vi "SUB_Write_GEN4_Init_data_V2_0_1.vi"(0 "Port-act 1":refnum<visa-resource-name>="COM8", 1 "data1":T7 {"Check sum" format="%x"; "Reserved_6" format="%x"; "Reserved_5" format="%x"; "Reserved_4" format="%x"; "Cal_Compart. A_10_4" format="%x"; "Reserved_3" format="%x"; "Reserved_2" format="%x"; "Reserved_1" format="%x"; "Cal_Compart. B_10_4" format="%x"; "Cal_Compart. B_10_3" format="%x"; "Cal_Compart. B_10_2" format="%x"; "Cal_Compart. B_10_1" format="%x"; "Cal_Compart. A_10_3" format="%x"; "Cal_Compart. A_10_2" format="%x"; "Cal_Compart. A_10_1" format="%x"; "Operative Side" format="%x"; "Firmware Revision" format="%x"; "Packet ID" format="%x"}, 2 "data2":T6 {"Check sum" format="%x"; "Cal_Compart. B_12_4" format="%x"; "Cal_Compart. B_12_3" format="%x"; "Cal_Compart. B_12_2" format="%x"; "Cal_Compart. B_11_2" format="%x"; "Cal_Compart. B_12_1" format="%x"; "Cal_Compart. A_12_4" format="%x"; "Cal_Compart. A_12_3" format="%x"; "Cal_Compart. A_12_2" format="%x"; "Cal_Compart. A_12_1" format="%x"; "Cal_Compart. B_11_4" format="%x"; "Cal_Compart. B_11_3" format="%x"; "Cal_Compart. B_11_1" format="%x"; "Cal_Compart. A_11_4" format="%x"; "Cal_Compart. A_11_3" format="%x"; "Cal_Compart. A_11_2" format="%x"; "Cal_Compart. A_11_1" format="%x"; "Packet ID" format="%x"}, 3 "Device information":T13 {"Check sum 2" format="%x"; "Device Type L" format="%x"; "Device Type H" format="%x"; "Check sum" format="%x"; "Scale B" format="%x"; "Scale A" format="%x"; "Manufacturer Lot ID 4" format="%x"; "Manufacturer Lot ID 3" format="%x"; "Manufacturer Lot ID 2" format="%x"; "Manufacturer Lot ID 1" format="%x"; "Day" format="%x"; "Month" format="%x"; "Year" format="%x"; "Device ID 4" format="%x"; "Device ID 3" format="%x"; "Device ID 2" format="%x"; "Device ID 1" format="%x"; "Packet ID" format="%x"}, 4 "Cal information":T12 {"Check sum" format="%x"; "Voltage L 2.8V" format="%x"; "Voltage H 2.8V" format="%x"; "Voltage L 3.1V" format="%x"; "Acc Z_L_Cal" format="%x"; "Voltage H 3.1V" format="%x"; "Gyro Z_L_Cal" format="%x"; "Gyro Z_H_Cal" format="%x"; "Gyro Y_L_Cal" format="%x"; "Gyro Y_H_Cal" format="%x"; "Gyro X_L_Cal" format="%x"; "Gyro X_H_Cal" format="%x"; "Acc Z_H_Cal" format="%x"; "Acc Y_L_Cal" format="%x"; "Acc Y_H_Cal" format="%x"; "Acc X_L_Cal" format="%x"; "Acc X_H_Cal" format="%x"; "Packet ID" format="%x"}, 5 "data3":T5 {"Check sum" format="%x"; "Cal_Compart. B_14_4" format="%x"; "Cal_Compart. B_14_3" format="%x"; "Cal_Compart. B_14_2" format="%x"; "Cal_Compart. B_13_2" format="%x"; "Cal_Compart. B_14_1" format="%x"; "Cal_Compart. A_14_4" format="%x"; "Cal_Compart. A_14_3" format="%x"; "Cal_Compart. A_14_2" format="%x"; "Cal_Compart. A_14_1" format="%x"; "Cal_Compart. B_13_4" format="%x"; "Cal_Compart. B_13_3" format="%x"; "Cal_Compart. B_13_1" format="%x"; "Cal_Compart. A_13_4" format="%x"; "Cal_Compart. A_13_3" format="%x"; "Cal_Compart. A_13_2" format="%x"; "Cal_Compart. A_13_1" format="%x"; "Packet ID" format="%x"}, 6 "data4":T4 {"Check sum" format="%x"; "Reserved_8" format="%x"; "Reserved_7" format="%x"; "Reserved_6" format="%x"; "Cal_Compart. B_16_2" format="%x"; "Reserved_5" format="%x"; "Reserved_4" format="%x"; "Reserved_3" format="%x"; "Reserved_2" format="%x"; "Reserved_1" format="%x"; "Cal_Compart. B_16_4" format="%x"; "Cal_Compart. B_16_3" format="%x"; "Cal_Compart. B_16_1" format="%x"; "Cal_Compart. A_16_4" format="%x"; "Cal_Compart. A_16_3" format="%x"; "Cal_Compart. A_16_2" format="%x"; "Cal_Compart. A_16_1" format="%x"; "Packet ID" format="%x"}, 7 "Connection Status":T8={"MAC Address"="F8:B8:54:EF:76:8D", "cnx handle"=0, "cnx flags"=5, "Address Type"=1, "Connection Interval (ms)"=8, "Timeout(ms)"=1000, "Latency"=0, "bonding handle"=255} {"Address Type" items=["Public", "Random"]}, 8 "Acclerometer value(0, 45)":T3 {"Check sum" format="%x"; "Reserved_4" format="%x"; "Reserved_3" format="%x"; "Reserved_2" format="%x"; "Acc. Z_0 val_L" format="%x"; "Reserved_1" format="%x"; "Acc. Z_45 val_L" format="%x"; "Acc. Z_45 val_H" format="%x"; "Acc. Y_45 val_L" format="%x"; "Acc. Y_45 val_H" format="%x"; "Acc. X_45 val_L" format="%x"; "Acc. X_45 val_H" format="%x"; "Acc. Z_0 val_H" format="%x"; "Acc. Y_0 val_L" format="%x"; "Acc. Y_0 val_H" format="%x"; "Acc. X_0 val_L" format="%x"; "Acc. X_0 val_H" format="%x"; "Packet ID" format="%x"}, 9 "Acclerometer value(90, 180)":T2 {"Check sum" format="%x"; "Reserved_2" format="%x"; "Reserved_1" format="%x"; "second counter_2" format="%x"; "Acc. Z_90 val_L" format="%x"; "second counter_1" format="%x"; "Acc. Z_180 val_L" format="%x"; "Acc. Z_180 val_H" format="%x"; "Acc. Y_180 val_L" format="%x"; "Acc. Y_180 val_H" format="%x"; "Acc. X_180 val_L" format="%x"; "Acc. X_180 val_H" format="%x"; "Acc. Z_90 val_H" format="%x"; "Acc. Y_90 val_L" format="%x"; "Acc. Y_90 val_H" format="%x"; "Acc. X_90 val_L" format="%x"; "Acc. X_90 val_H" format="%x"; "Packet ID" format="%x"}, 10 "배열":u8[](array[numeric]), 12 "Mode":T10, 13 "PCAP zero information":T11 {"Check sum" format="%x"; "Sensor 8_L" format="%x"; "Sensor 8_H" format="%x"; "Sensor 7_L" format="%x"; "Sensor 7_H" format="%x"; "Sensor 6_L" format="%x"; "Sensor 6_H" format="%x"; "Sensor 5_L" format="%x"; "Sensor 5_H" format="%x"; "Sensor 4_L" format="%x"; "Sensor 4_H" format="%x"; "Sensor 3_L" format="%x"; "Sensor 3_H" format="%x"; "Sensor 2_L" format="%x"; "Sensor 2_H" format="%x"; "Sensor 1_L" format="%x"; "Sensor 1_H" format="%x"; "Packet ID" format="%x"}, 14 "Interval Time":enum16{"10ms", "33ms", "50ms"}(ring)) -> (27 "불리언":bool)   [LabVIEW 2015]
uses:
  Cluster Type/Device information.ctl
  Cluster Type/Cal information.ctl
  Cluster Type/PCAP zero information.ctl
  Type definition/write_mode.ctl
  Lib_Bled112 toolkit/type_def/connection_status_bundle.ctl
  Lib_Bled112 toolkit/type_def/address_type.ctl
  Cluster Type/add data1.ctl
  Cluster Type/add data2.ctl
  Cluster Type/add data3.ctl
  Cluster Type/add data4.ctl
  Cluster Type/Acclerometer value(0, 45).ctl
  Cluster Type/Acclerometer value(90, 180).ctl
  Lib_Bled112 toolkit/ble_functions/ble_write_by_handle_uint8array.vi
panel:
  in  "열거형":T1(ring)
  in  "Delay(ms)":u32=3
  # "(Device Type is divided 1byte)"
  # "=> Sensor Offset Valure"
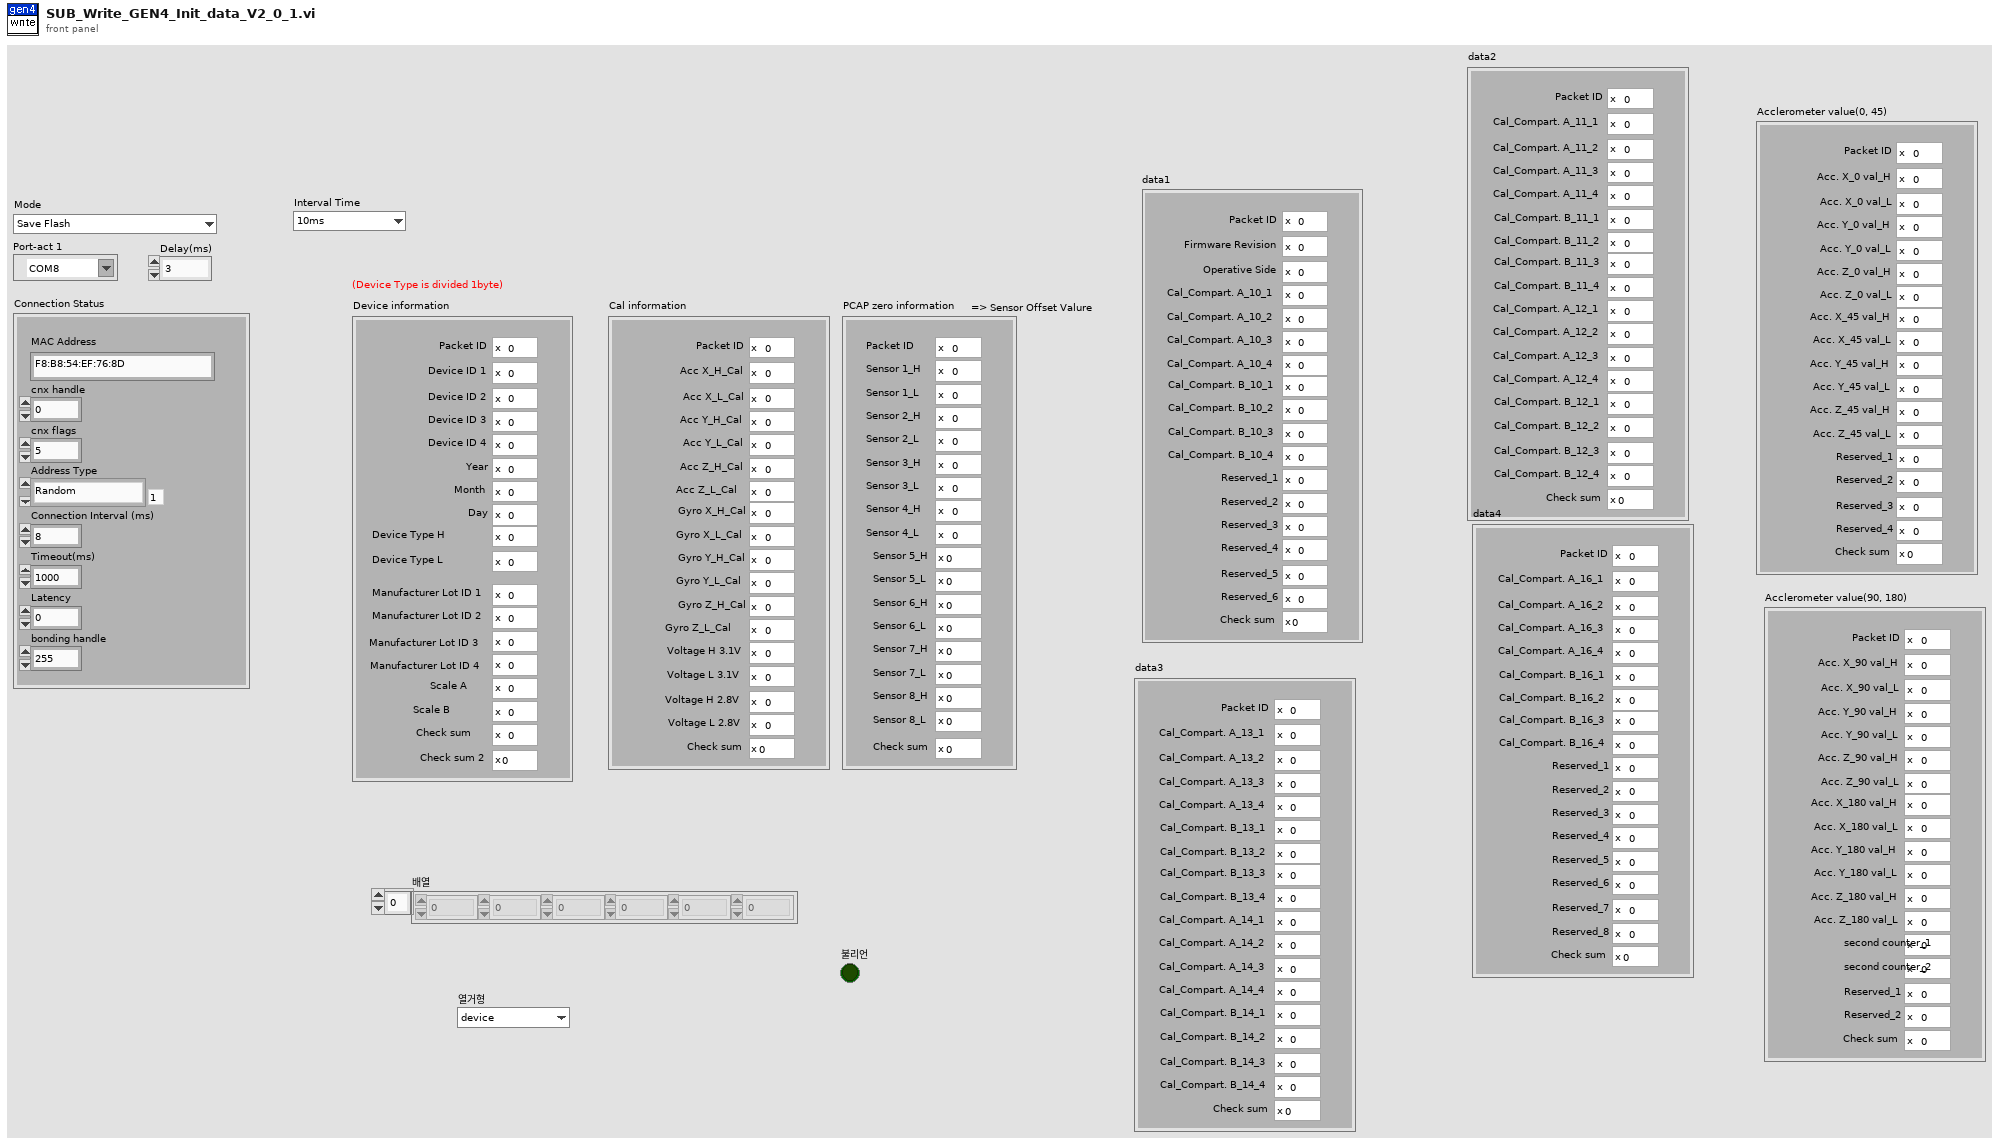
[diagram p1: front panel]
types:
  T1 = enum16{"device", "cal infor", "pcap", "data1", "data2", "data3", "data4", "acc 0", "acc 90", "42"}
  T2 = typedef "Acclerometer value(90, 180).ctl" = cluster{"Packet ID":u8, "Acc. X_90 val_H":u8, "Acc. X_90 val_L":u8, "Acc. Y_90 val_H":u8, "Acc. Y_90 val_L":u8, "Acc. Z_90 val_H":u8, "Acc. Z_90 val_L":u8, "Acc. X_180 val_H":u8, "Acc. X_180 val_L":u8, "Acc. Y_180 val_H":u8, "Acc. Y_180 val_L":u8, "Acc. Z_180 val_H":u8, "Acc. Z_180 val_L":u8, "second counter_1":u8, "second counter_2":u8, "Reserved_1":u8, "Reserved_2":u8, "Check sum":u8}
  T3 = typedef "Acclerometer value(0, 45).ctl" = cluster{"Packet ID":u8, "Acc. X_0 val_H":u8, "Acc. X_0 val_L":u8, "Acc. Y_0 val_H":u8, "Acc. Y_0 val_L":u8, "Acc. Z_0 val_H":u8, "Acc. Z_0 val_L":u8, "Acc. X_45 val_H":u8, "Acc. X_45 val_L":u8, "Acc. Y_45 val_H":u8, "Acc. Y_45 val_L":u8, "Acc. Z_45 val_H":u8, "Acc. Z_45 val_L":u8, "Reserved_1":u8, "Reserved_2":u8, "Reserved_3":u8, "Reserved_4":u8, "Check sum":u8}
  T4 = typedef "add data4.ctl" = cluster{"Packet ID":u8, "Cal_Compart. A_16_1":u8, "Cal_Compart. A_16_2":u8, "Cal_Compart. A_16_3":u8, "Cal_Compart. A_16_4":u8, "Cal_Compart. B_16_1":u8, "Cal_Compart. B_16_2":u8, "Cal_Compart. B_16_3":u8, "Cal_Compart. B_16_4":u8, "Reserved_1":u8, "Reserved_2":u8, "Reserved_3":u8, "Reserved_4":u8, "Reserved_5":u8, "Reserved_6":u8, "Reserved_7":u8, "Reserved_8":u8, "Check sum":u8}
  T5 = typedef "add data3.ctl" = cluster{"Packet ID":u8, "Cal_Compart. A_13_1":u8, "Cal_Compart. A_13_2":u8, "Cal_Compart. A_13_3":u8, "Cal_Compart. A_13_4":u8, "Cal_Compart. B_13_1":u8, "Cal_Compart. B_13_2":u8, "Cal_Compart. B_13_3":u8, "Cal_Compart. B_13_4":u8, "Cal_Compart. A_14_1":u8, "Cal_Compart. A_14_2":u8, "Cal_Compart. A_14_3":u8, "Cal_Compart. A_14_4":u8, "Cal_Compart. B_14_1":u8, "Cal_Compart. B_14_2":u8, "Cal_Compart. B_14_3":u8, "Cal_Compart. B_14_4":u8, "Check sum":u8}
  T6 = typedef "add data2.ctl" = cluster{"Packet ID":u8, "Cal_Compart. A_11_1":u8, "Cal_Compart. A_11_2":u8, "Cal_Compart. A_11_3":u8, "Cal_Compart. A_11_4":u8, "Cal_Compart. B_11_1":u8, "Cal_Compart. B_11_2":u8, "Cal_Compart. B_11_3":u8, "Cal_Compart. B_11_4":u8, "Cal_Compart. A_12_1":u8, "Cal_Compart. A_12_2":u8, "Cal_Compart. A_12_3":u8, "Cal_Compart. A_12_4":u8, "Cal_Compart. B_12_1":u8, "Cal_Compart. B_12_2":u8, "Cal_Compart. B_12_3":u8, "Cal_Compart. B_12_4":u8, "Check sum":u8}
  T7 = typedef "add data1.ctl" = cluster{"Packet ID":u8, "Firmware Revision":u8, "Operative Side":u8, "Cal_Compart. A_10_1":u8, "Cal_Compart. A_10_2":u8, "Cal_Compart. A_10_3":u8, "Cal_Compart. A_10_4":u8, "Cal_Compart. B_10_1":u8, "Cal_Compart. B_10_2":u8, "Cal_Compart. B_10_3":u8, "Cal_Compart. B_10_4":u8, "Reserved_1":u8, "Reserved_2":u8, "Reserved_3":u8, "Reserved_4":u8, "Reserved_5":u8, "Reserved_6":u8, "Check sum":u8}
  T8 = typedef "connection_status_bundle.ctl" = cluster{"MAC Address":string, "cnx handle":u8, "cnx flags":u8, "Address Type":T9, "Connection Interval (ms)":u16, "Timeout(ms)":u16, "Latency":u16, "bonding handle":u8}
  T9 = typedef "address_type.ctl" = u8
  T10 = typedef "write_mode.ctl" = enum16{"Save Flash", "Visa save", "Interval Change"}
  T11 = typedef "PCAP zero information.ctl" = cluster{"Packet ID":u8, "Sensor 1_H":u8, "Sensor 1_L":u8, "Sensor 2_H":u8, "Sensor 2_L ":u8, "Sensor 3_H":u8, "Sensor 3_L":u8, "Sensor 4_H":u8, "Sensor 4_L":u8, "Sensor 5_H":u8, "Sensor 5_L":u8, "Sensor 6_H":u8, "Sensor 6_L":u8, "Sensor 7_H":u8, "Sensor 7_L":u8, "Sensor 8_H":u8, "Sensor 8_L":u8, "Check sum":u8}
  T12 = typedef "Cal information.ctl" = cluster{"Packet ID":u8, "Acc X_H_Cal":u8, "Acc X_L_Cal":u8, "Acc Y_H_Cal":u8, "Acc Y_L_Cal":u8, "Acc Z_H_Cal":u8, "Acc Z_L_Cal":u8, "Gyro X_H_Cal":u8, "Gyro X_L_Cal":u8, "Gyro Y_H_Cal":u8, "Gyro Y_L_Cal":u8, "Gyro Z_H_Cal":u8, "Gyro Z_L_Cal":u8, "Voltage H 3.1V":u8, "Voltage L 3.1V":u8, "Voltage H 2.8V":u8, "Voltage L 2.8V":u8, "Check sum":u8}
  T13 = typedef "Device information.ctl" = cluster{"Packet ID":u8, "Device ID 1":u8, "Device ID 2":u8, "Device ID 3":u8, "Device ID 4":u8, "Year":u8, "Month":u8, "Day":u8, "Device Type H":u8, "Device Type L":u8, "Manufacturer Lot ID 1":u8, "Manufacturer Lot ID 2":u8, "Manufacturer Lot ID 3":u8, "Manufacturer Lot ID 4":u8, "Scale A":u8, "Scale B":u8, "Check sum":u8, "Check sum 2":u8}
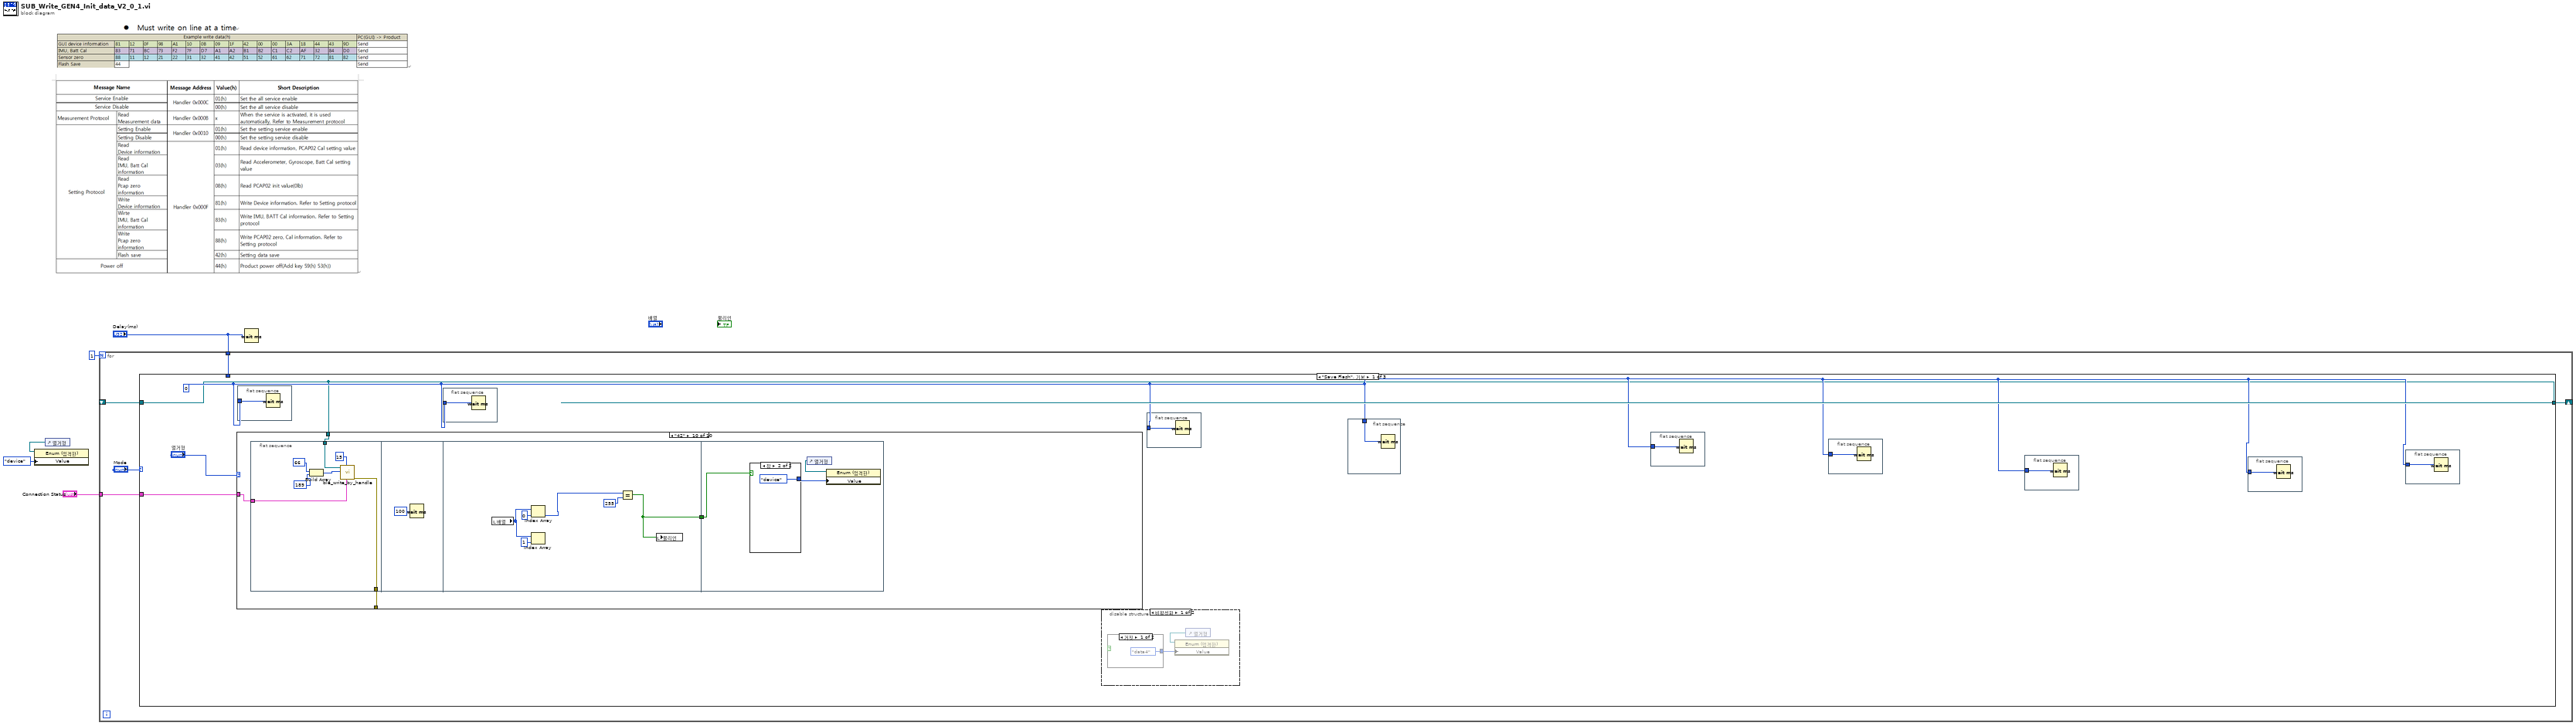
[diagram p0: block diagram]
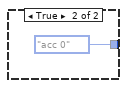
[diagram p2: hidden frame]
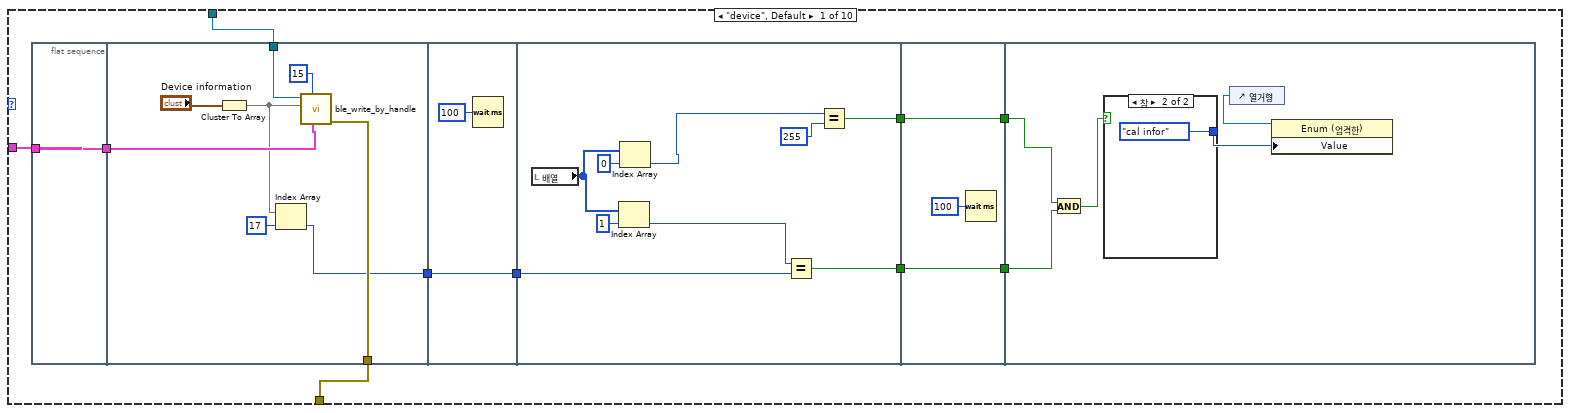
[diagram p4: hidden frame]
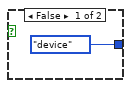
[diagram p5: hidden frame]
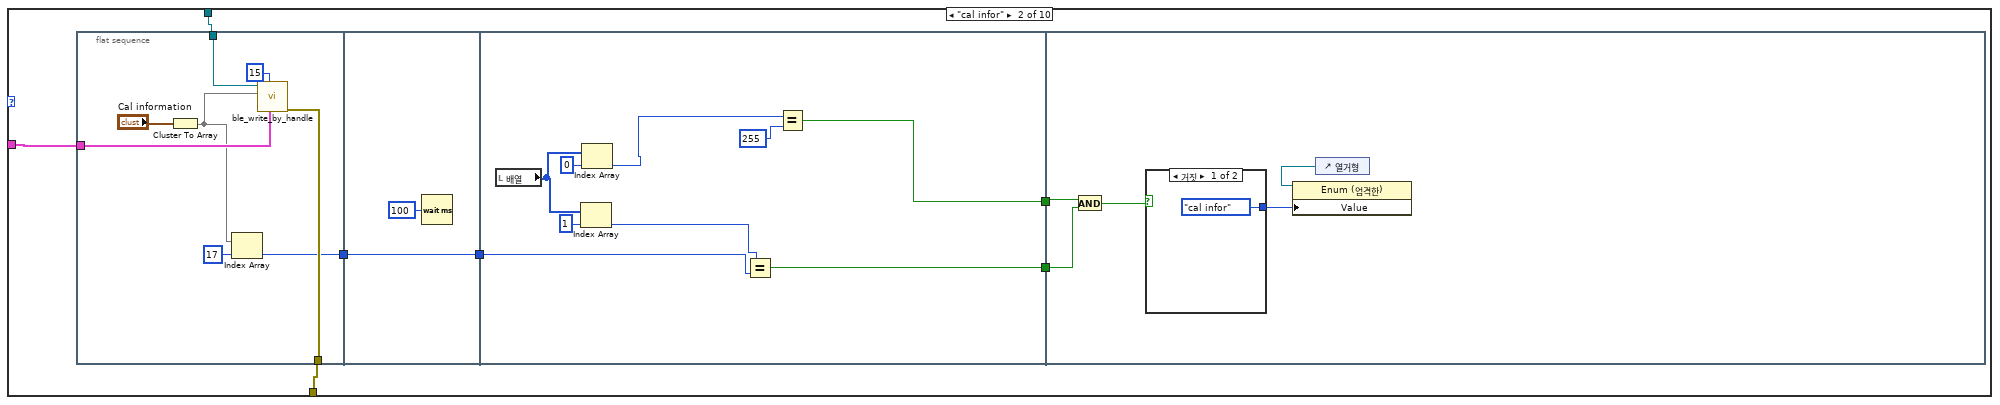
[diagram p6: hidden frame]
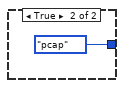
[diagram p7: hidden frame]
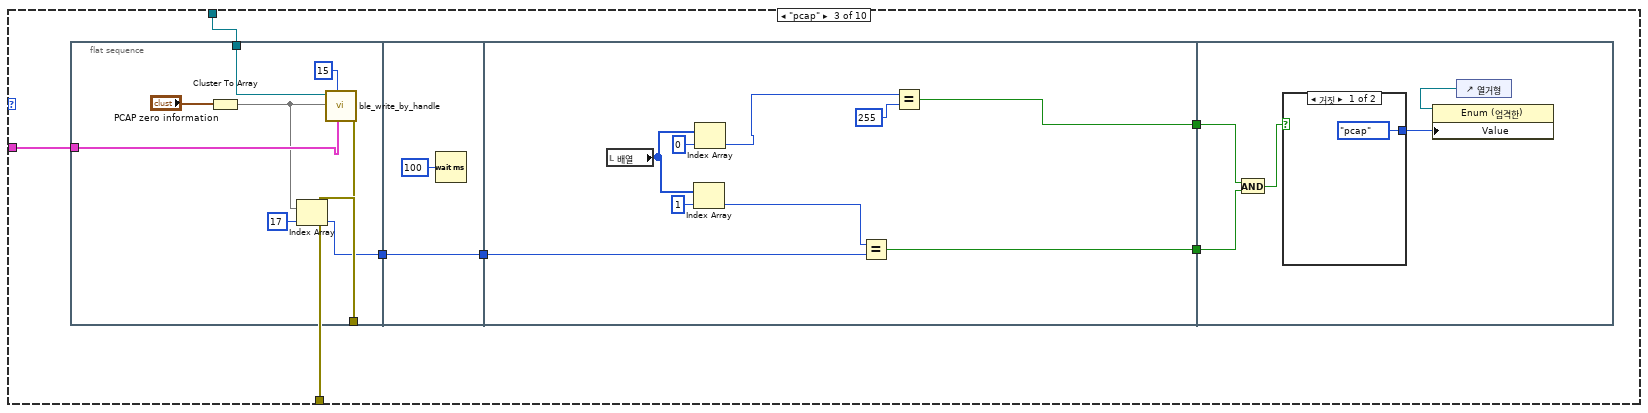
[diagram p8: hidden frame]
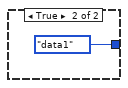
[diagram p9: hidden frame]
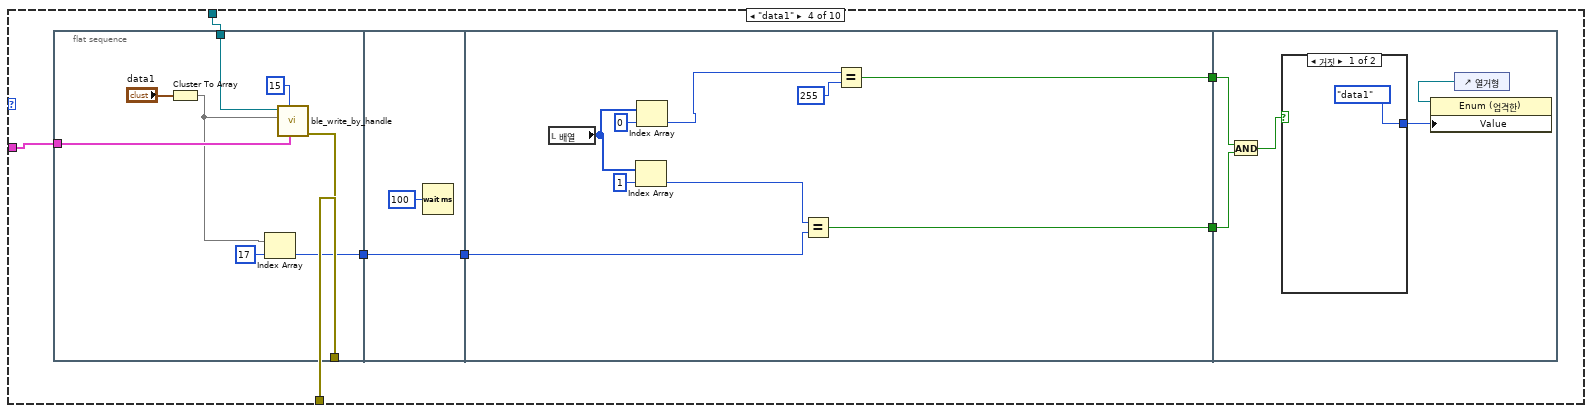
[diagram p10: hidden frame]
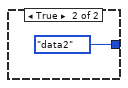
[diagram p11: hidden frame]
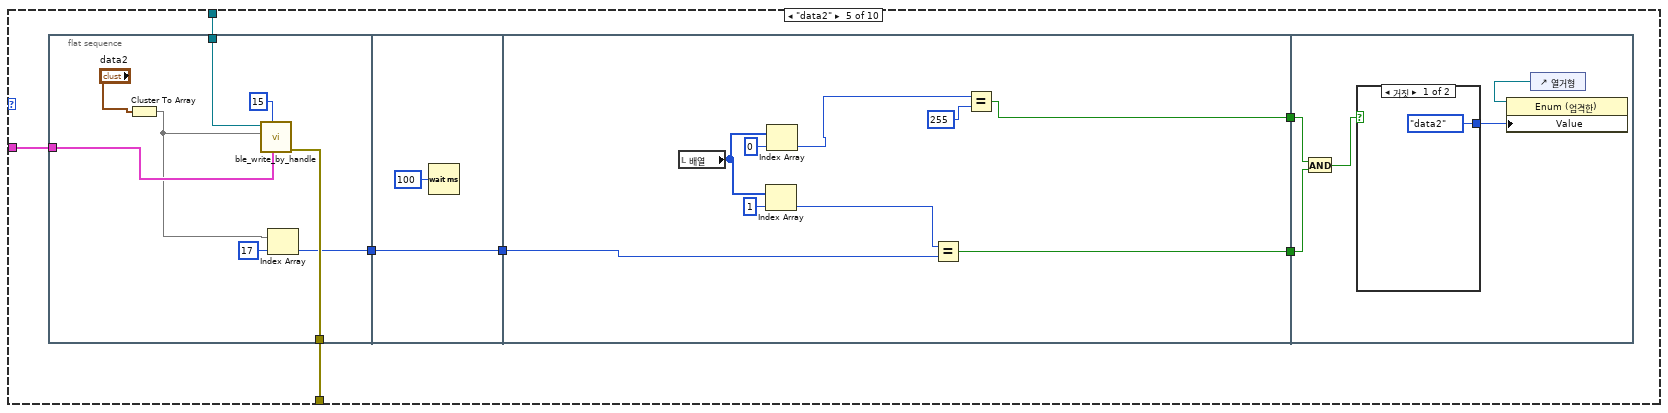
[diagram p12: hidden frame]
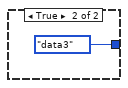
[diagram p13: hidden frame]
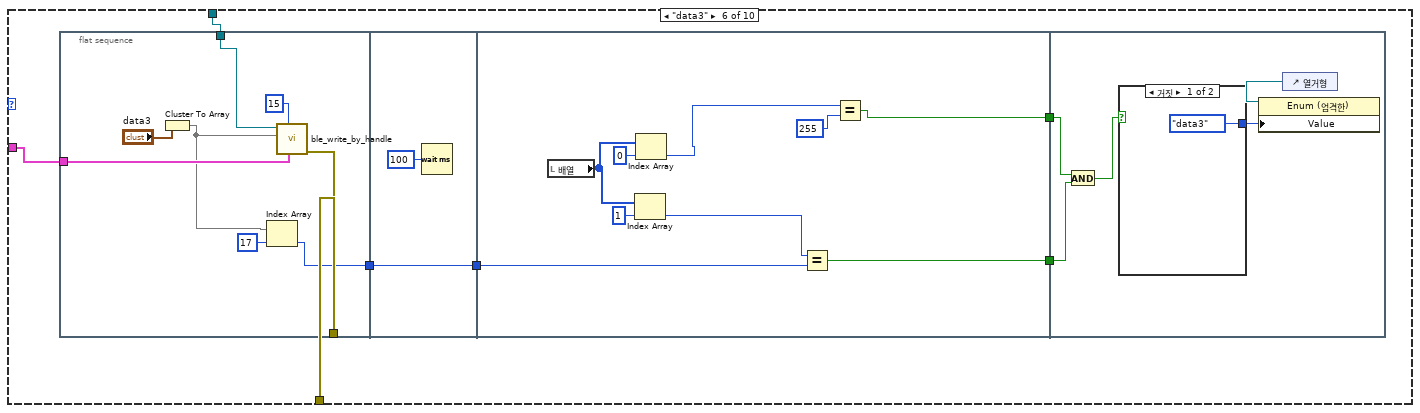
[diagram p14: hidden frame]
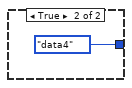
[diagram p15: hidden frame]
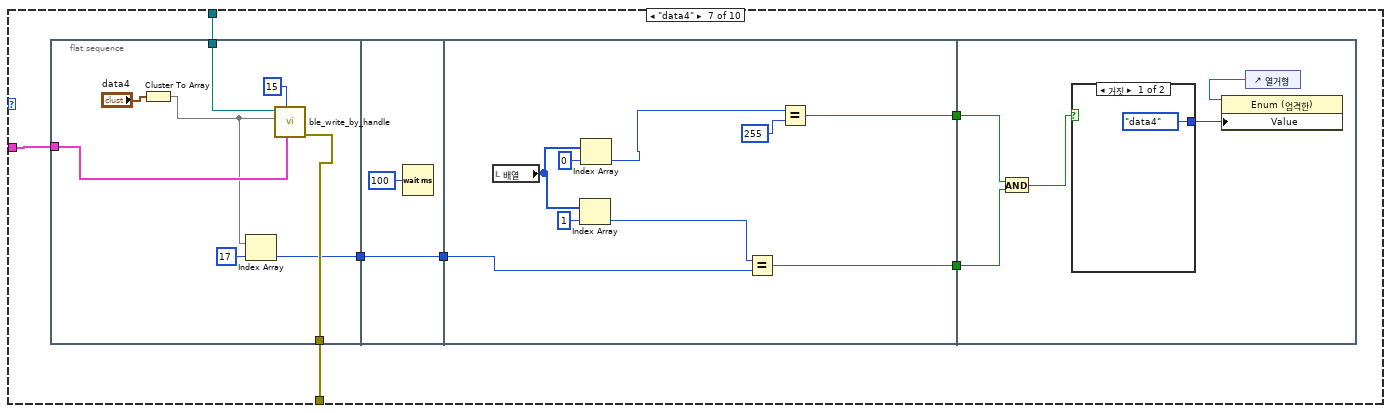
[diagram p16: hidden frame]
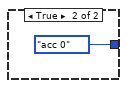
[diagram p17: hidden frame]
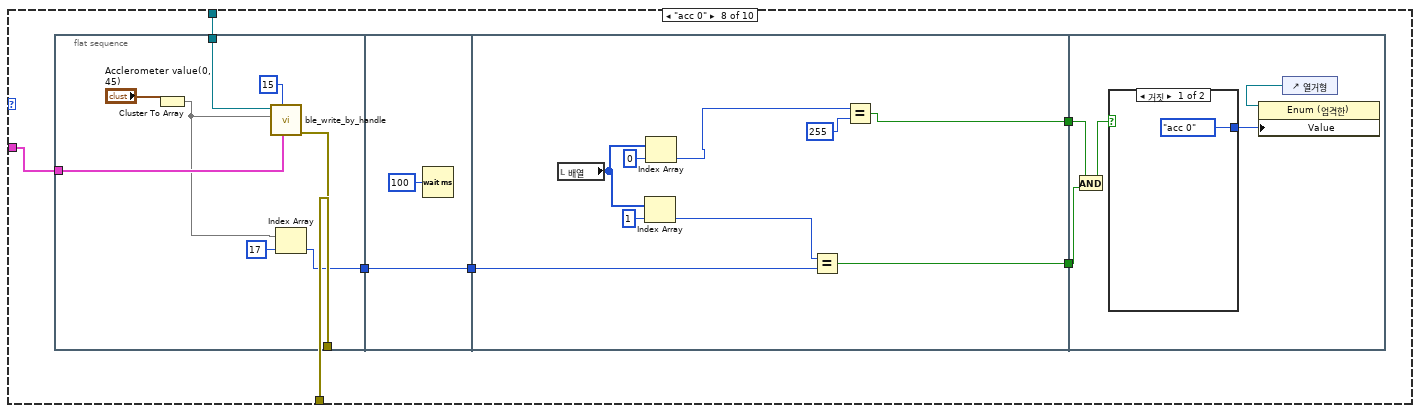
[diagram p18: hidden frame]
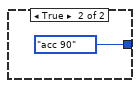
[diagram p19: hidden frame]
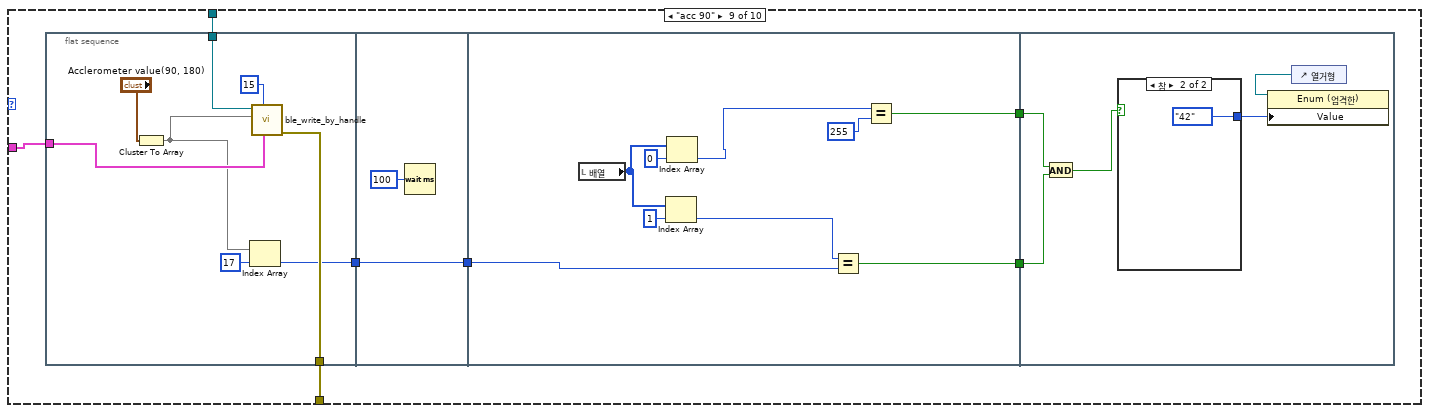
[diagram p20: hidden frame]
diagram:
  n1 = control-ref of="열거형"() -> (w1:refnum<vi>)
  n2 = property class="Enum (엄격한)"(reference=w1, "Value"=T1."device" ("값")) -> ()  [unwired: 1 in, 2 out]
  n3 = for {
    N: 1 -> [_]
    shift-right: [w9] -> _
    shift-left: _ -> [w8]
    tunnel: "Connection Status" -> [w7]
    tunnel: "Delay(ms)" -> [w6]
    n4 = case shown="\"Save Flash\", 기본" "Mode" {
      tunnel: [w11 w372 "Port-act 1"] -> w9
      tunnel: w8 -> [w11 w372 _]
      tunnel: w7 -> [w12 w385 _]
      tunnel: w6 -> [_ w360 _]
      frame "Save Flash", Default {
        w14 = u32 0 ("대기 시간(ms)")
        n5 = case shown="\"42\"" "열거형" {
          tunnel: w12 -> [w28 w64 w98 w130 w164 w196 w230 w263 w296 w326]
          tunnel: w11 -> [w27 w65 w97 w131 w163 w197 w229 w262 w295 w325]
          tunnel: [w26 w63 w96 w129 w162 w195 w228 w261 w294 w324] -> _
          frame "device", Default {
            n6 = flat-sequence {
              tunnel: w28 -> [w29]
              tunnel: [w29] -> w25
              tunnel: w27 -> [w34]
              tunnel: [w33] -> w26
              tunnel: w25 -> [w35]
              tunnel: [w30] -> w22
              tunnel: w22 -> [w38]
              tunnel: [w38] -> w21
              tunnel: [w43] -> w24
              tunnel: w21 -> [w41]
              tunnel: [w40] -> w20
              tunnel: w24 -> [w51]
              tunnel: [w51] -> w23
              tunnel: w20 -> [w49]
              tunnel: [w49] -> w19
              tunnel: w23 -> [w54]
              tunnel: w19 -> [w53]
              frame #0 {
              }
              frame #1 {
                n7 = Cluster To Array(cluster="Device information") -> (array=w31:u8[])
                n8 = Index Array(array=w31, index=17 ("인덱스")) -> (element=w30:u8)
                n9 = call-poly "ble_write_by_handle.vi"("Connection Status"=w35, "Handle"=u16 15, "data (uint8array)"=w31, "COM Bluegiga in"=w34) -> ("error out"=w33:errorcluster)  [unwired: 6 in, 1 out]
              }
              frame #2 {
                n10 = Wait (ms)(milliseconds to wait=u32 100 ("대기 시간(ms)")) -> ()  [unwired: 1 out]
              }
              frame #3 {
                n11 = local read "배열"() -> (w44:u8[])
                n12 = Index Array(array=w44, index=1 ("인덱스")) -> (element=w42:u8)
                n13 = Index Array(array=w44, index=0 ("인덱스")) -> (element=w47:u8)
                n14 = Equal?(x=w42, y=w41) -> (x = y?=w40:bool)
                n15 = Equal?(x=w47, y=u8 255) -> (x = y?=w43:bool)
              }
              frame #4 {
                n16 = Wait (ms)(milliseconds to wait=u32 100 ("대기 시간(ms)")) -> ()  [unwired: 1 out]
              }
              frame #5 {
                n17 = And(x=w54, y=w53) -> (x .and. y?=w52:bool)
                n18 = case shown="참" w52 {
                  tunnel: [T1."device" ("값") T1."cal infor" ("값")] -> w55
                  frame False {
                  }
                  frame True {
                  }
                }
                n19 = control-ref of="열거형"() -> (w56:refnum<vi>)
                n20 = property class="Enum (엄격한)"(reference=w56, "Value"=w55) -> ()  [unwired: 1 in, 2 out]
              }
            }
          }
          frame "cal infor" {
            n21 = flat-sequence {
              tunnel: w65 -> [w71]
              tunnel: w64 -> [w70]
              tunnel: [w69] -> w63
              tunnel: [w66] -> w61
              tunnel: w61 -> [w74]
              tunnel: [w74] -> w60
              tunnel: [w79] -> w62
              tunnel: w60 -> [w78]
              tunnel: [w76] -> w59
              tunnel: w62 -> [w87]
              tunnel: w59 -> [w86]
              frame #0 {
                n22 = Cluster To Array(cluster="Cal information") -> (array=w67:u8[])
                n23 = Index Array(array=w67, index=17 ("인덱스")) -> (element=w66:u8)
                n24 = call-poly "ble_write_by_handle.vi"("Connection Status"=w70, "Handle"=u16 15, "data (uint8array)"=w67, "COM Bluegiga in"=w71) -> ("error out"=w69:errorcluster)  [unwired: 6 in, 1 out]
              }
              frame #1 {
                n25 = Wait (ms)(milliseconds to wait=u32 100 ("대기 시간(ms)")) -> ()  [unwired: 1 out]
              }
              frame #2 {
                n26 = local read "배열"() -> (w80:u8[])
                n27 = Index Array(array=w80, index=1 ("인덱스")) -> (element=w77:u8)
                n28 = Index Array(array=w80, index=0 ("인덱스")) -> (element=w83:u8)
                n29 = Equal?(x=w77, y=w78) -> (x = y?=w76:bool)
                n30 = Equal?(x=w83, y=u8 255) -> (x = y?=w79:bool)
              }
              frame #3 {
                n31 = And(x=w87, y=w86) -> (x .and. y?=w85:bool)
                n32 = case shown="거짓" w85 {
                  tunnel: [T1."cal infor" ("값") T1."pcap" ("값")] -> w88
                  frame False {
                  }
                  frame True {
                  }
                }
                n33 = control-ref of="열거형"() -> (w89:refnum<vi>)
                n34 = property class="Enum (엄격한)"(reference=w89, "Value"=w88) -> ()  [unwired: 1 in, 2 out]
              }
            }
          }
          frame "pcap" {
            n35 = flat-sequence {
              tunnel: w98 -> [w104]
              tunnel: w97 -> [w103]
              tunnel: [w102] -> w96
              tunnel: [w99] -> w94
              tunnel: w94 -> [w107]
              tunnel: [w107] -> w93
              tunnel: [w112] -> w95
              tunnel: w93 -> [w110]
              tunnel: [w109] -> w92
              tunnel: w95 -> [w120]
              tunnel: w92 -> [w119]
              frame #0 {
                n36 = Cluster To Array(cluster="PCAP zero information") -> (array=w100:u8[])
                n37 = Index Array(array=w100, index=17 ("인덱스")) -> (element=w99:u8)
                n38 = call-poly "ble_write_by_handle.vi"("Connection Status"=w104, "Handle"=u16 15, "data (uint8array)"=w100, "COM Bluegiga in"=w103) -> ("error out"=w102:errorcluster)  [unwired: 6 in, 1 out]
              }
              frame #1 {
                n39 = Wait (ms)(milliseconds to wait=u32 100 ("대기 시간(ms)")) -> ()  [unwired: 1 out]
              }
              frame #2 {
                n40 = local read "배열"() -> (w113:u8[])
                n41 = Index Array(array=w113, index=1 ("인덱스")) -> (element=w111:u8)
                n42 = Index Array(array=w113, index=0 ("인덱스")) -> (element=w116:u8)
                n43 = Equal?(x=w111, y=w110) -> (x = y?=w109:bool)
                n44 = Equal?(x=w116, y=u8 255) -> (x = y?=w112:bool)
              }
              frame #3 {
                n45 = And(x=w120, y=w119) -> (x .and. y?=w118:bool)
                n46 = case shown="거짓" w118 {
                  tunnel: [T1."pcap" ("값") T1."data1" ("값")] -> w121
                  frame False {
                  }
                  frame True {
                  }
                }
                n47 = control-ref of="열거형"() -> (w122:refnum<vi>)
                n48 = property class="Enum (엄격한)"(reference=w122, "Value"=w121) -> ()  [unwired: 1 in, 2 out]
              }
            }
          }
          frame "data1" {
            n49 = flat-sequence {
              tunnel: w131 -> [w137]
              tunnel: w130 -> [w136]
              tunnel: [w135] -> w129
              tunnel: [w132] -> w127
              tunnel: w127 -> [w140]
              tunnel: [w140] -> w126
              tunnel: [w145] -> w128
              tunnel: w126 -> [w144]
              tunnel: [w142] -> w125
              tunnel: w128 -> [w153]
              tunnel: w125 -> [w152]
              frame #0 {
                n50 = Cluster To Array(cluster="data1") -> (array=w133:u8[])
                n51 = Index Array(array=w133, index=17 ("인덱스")) -> (element=w132:u8)
                n52 = call-poly "ble_write_by_handle.vi"("Connection Status"=w136, "Handle"=u16 15, "data (uint8array)"=w133, "COM Bluegiga in"=w137) -> ("error out"=w135:errorcluster)  [unwired: 6 in, 1 out]
              }
              frame #1 {
                n53 = Wait (ms)(milliseconds to wait=u32 100 ("대기 시간(ms)")) -> ()  [unwired: 1 out]
              }
              frame #2 {
                n54 = local read "배열"() -> (w146:u8[])
                n55 = Index Array(array=w146, index=1 ("인덱스")) -> (element=w143:u8)
                n56 = Index Array(array=w146, index=0 ("인덱스")) -> (element=w149:u8)
                n57 = Equal?(x=w143, y=w144) -> (x = y?=w142:bool)
                n58 = Equal?(x=w149, y=u8 255) -> (x = y?=w145:bool)
              }
              frame #3 {
                n59 = And(x=w153, y=w152) -> (x .and. y?=w151:bool)
                n60 = case shown="거짓" w151 {
                  tunnel: [T1."data1" ("값") T1."data2" ("값")] -> w154
                  frame False {
                  }
                  frame True {
                  }
                }
                n61 = control-ref of="열거형"() -> (w155:refnum<vi>)
                n62 = property class="Enum (엄격한)"(reference=w155, "Value"=w154) -> ()  [unwired: 1 in, 2 out]
              }
            }
          }
          frame "data2" {
            n63 = flat-sequence {
              tunnel: w164 -> [w170]
              tunnel: w163 -> [w169]
              tunnel: [w168] -> w162
              tunnel: [w165] -> w160
              tunnel: w160 -> [w173]
              tunnel: [w173] -> w159
              tunnel: [w178] -> w161
              tunnel: w159 -> [w176]
              tunnel: [w175] -> w158
              tunnel: w161 -> [w186]
              tunnel: w158 -> [w185]
              frame #0 {
                n64 = Cluster To Array(cluster="data2") -> (array=w166:u8[])
                n65 = call-poly "ble_write_by_handle.vi"("Connection Status"=w170, "Handle"=u16 15, "data (uint8array)"=w166, "COM Bluegiga in"=w169) -> ("error out"=w168:errorcluster)  [unwired: 6 in, 1 out]
                n66 = Index Array(array=w166, index=17 ("인덱스")) -> (element=w165:u8)
              }
              frame #1 {
                n67 = Wait (ms)(milliseconds to wait=u32 100 ("대기 시간(ms)")) -> ()  [unwired: 1 out]
              }
              frame #2 {
                n68 = local read "배열"() -> (w179:u8[])
                n69 = Index Array(array=w179, index=1 ("인덱스")) -> (element=w177:u8)
                n70 = Index Array(array=w179, index=0 ("인덱스")) -> (element=w182:u8)
                n71 = Equal?(x=w177, y=w176) -> (x = y?=w175:bool)
                n72 = Equal?(x=w182, y=u8 255) -> (x = y?=w178:bool)
              }
              frame #3 {
                n73 = And(x=w186, y=w185) -> (x .and. y?=w184:bool)
                n74 = case shown="거짓" w184 {
                  tunnel: [T1."data2" ("값") T1."data3" ("값")] -> w187
                  frame False {
                  }
                  frame True {
                  }
                }
                n75 = control-ref of="열거형"() -> (w188:refnum<vi>)
                n76 = property class="Enum (엄격한)"(reference=w188, "Value"=w187) -> ()  [unwired: 1 in, 2 out]
              }
            }
          }
          frame "data3" {
            n77 = flat-sequence {
              tunnel: w197 -> [w203]
              tunnel: w196 -> [w202]
              tunnel: [w201] -> w195
              tunnel: [w198] -> w193
              tunnel: w193 -> [w206]
              tunnel: [w206] -> w192
              tunnel: [w211] -> w194
              tunnel: w192 -> [w209]
              tunnel: [w208] -> w191
              tunnel: w194 -> [w219]
              tunnel: w191 -> [w218]
              frame #0 {
                n78 = Cluster To Array(cluster="data3") -> (array=w199:u8[])
                n79 = Index Array(array=w199, index=17 ("인덱스")) -> (element=w198:u8)
                n80 = call-poly "ble_write_by_handle.vi"("Connection Status"=w202, "Handle"=u16 15, "data (uint8array)"=w199, "COM Bluegiga in"=w203) -> ("error out"=w201:errorcluster)  [unwired: 6 in, 1 out]
              }
              frame #1 {
                n81 = Wait (ms)(milliseconds to wait=u32 100 ("대기 시간(ms)")) -> ()  [unwired: 1 out]
              }
              frame #2 {
                n82 = local read "배열"() -> (w212:u8[])
                n83 = Index Array(array=w212, index=1 ("인덱스")) -> (element=w210:u8)
                n84 = Index Array(array=w212, index=0 ("인덱스")) -> (element=w215:u8)
                n85 = Equal?(x=w210, y=w209) -> (x = y?=w208:bool)
                n86 = Equal?(x=w215, y=u8 255) -> (x = y?=w211:bool)
              }
              frame #3 {
                n87 = And(x=w219, y=w218) -> (x .and. y?=w217:bool)
                n88 = case shown="거짓" w217 {
                  tunnel: [T1."data3" ("값") T1."data4" ("값")] -> w220
                  frame False {
                  }
                  frame True {
                  }
                }
                n89 = control-ref of="열거형"() -> (w221:refnum<vi>)
                n90 = property class="Enum (엄격한)"(reference=w221, "Value"=w220) -> ()  [unwired: 1 in, 2 out]
              }
            }
          }
          frame "data4" {
            n91 = flat-sequence {
              tunnel: w230 -> [w236]
              tunnel: w229 -> [w235]
              tunnel: [w234] -> w228
              tunnel: [w232] -> w226
              tunnel: w226 -> [w239]
              tunnel: [w239] -> w225
              tunnel: [w244] -> w227
              tunnel: w225 -> [w242]
              tunnel: [w241] -> w224
              tunnel: w227 -> [w252]
              tunnel: w224 -> [w251]
              frame #0 {
                n92 = Cluster To Array(cluster="data4") -> (array=w231:u8[])
                n93 = Index Array(array=w231, index=17 ("인덱스")) -> (element=w232:u8)
                n94 = call-poly "ble_write_by_handle.vi"("Connection Status"=w236, "Handle"=u16 15, "data (uint8array)"=w231, "COM Bluegiga in"=w235) -> ("error out"=w234:errorcluster)  [unwired: 6 in, 1 out]
              }
              frame #1 {
                n95 = Wait (ms)(milliseconds to wait=u32 100 ("대기 시간(ms)")) -> ()  [unwired: 1 out]
              }
              frame #2 {
                n96 = local read "배열"() -> (w245:u8[])
                n97 = Index Array(array=w245, index=1 ("인덱스")) -> (element=w243:u8)
                n98 = Index Array(array=w245, index=0 ("인덱스")) -> (element=w248:u8)
                n99 = Equal?(x=w243, y=w242) -> (x = y?=w241:bool)
                n100 = Equal?(x=w248, y=u8 255) -> (x = y?=w244:bool)
              }
              frame #3 {
                n101 = And(x=w252, y=w251) -> (x .and. y?=w250:bool)
                n102 = case shown="거짓" w250 {
                  tunnel: [T1."data4" ("값") T1."acc 0" ("값")] -> w253
                  frame False {
                  }
                  frame True {
                  }
                }
                n103 = control-ref of="열거형"() -> (w254:refnum<vi>)
                n104 = property class="Enum (엄격한)"(reference=w254, "Value"=w253) -> ()  [unwired: 1 in, 2 out]
              }
            }
          }
          frame "acc 0" {
            n105 = flat-sequence {
              tunnel: w263 -> [w269]
              tunnel: w262 -> [w268]
              tunnel: [w267] -> w261
              tunnel: [w265] -> w259
              tunnel: w259 -> [w272]
              tunnel: [w272] -> w258
              tunnel: [w277] -> w260
              tunnel: w258 -> [w275]
              tunnel: [w274] -> w257
              tunnel: w260 -> [w285]
              tunnel: w257 -> [w284]
              frame #0 {
                n106 = Cluster To Array(cluster="Acclerometer value(0, 45)") -> (array=w264:u8[])
                n107 = call-poly "ble_write_by_handle.vi"("Connection Status"=w269, "Handle"=u16 15, "data (uint8array)"=w264, "COM Bluegiga in"=w268) -> ("error out"=w267:errorcluster)  [unwired: 6 in, 1 out]
                n108 = Index Array(array=w264, index=17 ("인덱스")) -> (element=w265:u8)
              }
              frame #1 {
                n109 = Wait (ms)(milliseconds to wait=u32 100 ("대기 시간(ms)")) -> ()  [unwired: 1 out]
              }
              frame #2 {
                n110 = local read "배열"() -> (w278:u8[])
                n111 = Index Array(array=w278, index=1 ("인덱스")) -> (element=w276:u8)
                n112 = Index Array(array=w278, index=0 ("인덱스")) -> (element=w281:u8)
                n113 = Equal?(x=w276, y=w275) -> (x = y?=w274:bool)
                n114 = Equal?(x=w281, y=u8 255) -> (x = y?=w277:bool)
              }
              frame #3 {
                n115 = And(x=w285, y=w284) -> (x .and. y?=w283:bool)
                n116 = case shown="거짓" w283 {
                  tunnel: [T1."acc 0" ("값") T1."acc 90" ("값")] -> w286
                  frame False {
                  }
                  frame True {
                  }
                }
                n117 = control-ref of="열거형"() -> (w287:refnum<vi>)
                n118 = property class="Enum (엄격한)"(reference=w287, "Value"=w286) -> ()  [unwired: 1 in, 2 out]
              }
            }
          }
          frame "acc 90" {
            n119 = flat-sequence {
              tunnel: w296 -> [w302]
              tunnel: w295 -> [w301]
              tunnel: [w300] -> w294
              tunnel: [w297] -> w292
              tunnel: w292 -> [w305]
              tunnel: [w305] -> w291
              tunnel: [w310] -> w293
              tunnel: w291 -> [w308]
              tunnel: [w307] -> w290
              tunnel: w293 -> [w318]
              tunnel: w290 -> [w317]
              frame #0 {
                n120 = Cluster To Array(cluster="Acclerometer value(90, 180)") -> (array=w298:u8[])
                n121 = Index Array(array=w298, index=17 ("인덱스")) -> (element=w297:u8)
                n122 = call-poly "ble_write_by_handle.vi"("Connection Status"=w302, "Handle"=u16 15, "data (uint8array)"=w298, "COM Bluegiga in"=w301) -> ("error out"=w300:errorcluster)  [unwired: 6 in, 1 out]
              }
              frame #1 {
                n123 = Wait (ms)(milliseconds to wait=u32 100 ("대기 시간(ms)")) -> ()  [unwired: 1 out]
              }
              frame #2 {
                n124 = local read "배열"() -> (w311:u8[])
                n125 = Index Array(array=w311, index=1 ("인덱스")) -> (element=w309:u8)
                n126 = Index Array(array=w311, index=0 ("인덱스")) -> (element=w314:u8)
                n127 = Equal?(x=w309, y=w308) -> (x = y?=w307:bool)
                n128 = Equal?(x=w314, y=u8 255) -> (x = y?=w310:bool)
              }
              frame #3 {
                n129 = And(x=w318, y=w317) -> (x .and. y?=w316:bool)
                n130 = case shown="참" w316 {
                  tunnel: [T1."acc 90" ("값") T1."42" ("값")] -> w319
                  frame False {
                  }
                  frame True {
                  }
                }
                n131 = control-ref of="열거형"() -> (w320:refnum<vi>)
                n132 = property class="Enum (엄격한)"(reference=w320, "Value"=w319) -> ()  [unwired: 1 in, 2 out]
              }
            }
          }
          frame "42" {
            n133 = flat-sequence {
              tunnel: w326 -> [w329]
              tunnel: w325 -> [w328]
              tunnel: [w327] -> w324
              tunnel: [w335] -> w323
              tunnel: w323 -> [w341]
              frame #0 {
                n134 = Build Array(u16 66 ("Handle"), u16 189 ("Handle")) -> (w332:u16[])
                n135 = call-poly "ble_write_by_handle.vi"("Connection Status"=w329, "Handle"=u16 15, "data (uint8array)"=w332, "COM Bluegiga in"=w328) -> ("error out"=w327:errorcluster)  [unwired: 6 in, 1 out]
              }
              frame #1 {
                n136 = Wait (ms)(milliseconds to wait=u32 100 ("대기 시간(ms)")) -> ()  [unwired: 1 out]
              }
              frame #2 {
                n137 = local read "배열"() -> (w336:u8[])
                n138 = Index Array(array=w336, index=1 ("인덱스")) -> ()  [unwired: 1 out]
                n139 = Index Array(array=w336, index=0 ("인덱스")) -> (element=w339:u8)
                n140 = Equal?(x=w339, y=u8 255) -> (x = y?=w335:bool)
                n141 = local write "불리언"(w335) -> ()
              }
              frame #3 {
                n142 = case shown="참" w341 {
                  tunnel: [T1."42" ("값") T1."device" ("값")] -> w342
                  frame False {
                  }
                  frame True {
                  }
                }
                n143 = control-ref of="열거형"() -> (w343:refnum<vi>)
                n144 = property class="Enum (엄격한)"(reference=w343, "Value"=w342) -> ()  [unwired: 1 in, 2 out]
              }
            }
          }
        }
        n145 = flat-sequence {
          tunnel: w14 -> [w353]
          frame #0 {
            n146 = Wait (ms)(milliseconds to wait=w353) -> ()  [unwired: 1 out]
          }
        }
        n147 = flat-sequence {
          tunnel: w14 -> [w352]
          frame #0 {
            n148 = Wait (ms)(milliseconds to wait=w352) -> ()  [unwired: 1 out]
          }
        }
        n149 = disable-structure shown="비활성화" {
          frame Disabled {
            n150 = case shown="거짓" {
              selector: _ -> [_ _]
              tunnel: [T1."data4" ("값") T1."acc 0" ("값")] -> w16
              frame False {
              }
              frame True {
              }
            }
            n151 = control-ref of="열거형"() -> (w15:refnum<vi>)
            n152 = property class="Enum (엄격한)"(reference=w15, "Value"=w16) -> ()  [unwired: 1 in, 2 out]
          }
          frame Enabled {
          }
        }
        n153 = flat-sequence {
          tunnel: w14 -> [w351]
          frame #0 {
            n154 = Wait (ms)(milliseconds to wait=w351) -> ()  [unwired: 1 out]
          }
        }
        n155 = flat-sequence {
          tunnel: w14 -> [w354]
          frame #0 {
            n156 = Wait (ms)(milliseconds to wait=w354) -> ()  [unwired: 1 out]
          }
        }
        n157 = flat-sequence {
          tunnel: w14 -> [w350]
          frame #0 {
            n158 = Wait (ms)(milliseconds to wait=w350) -> ()  [unwired: 1 out]
          }
        }
        n159 = flat-sequence {
          tunnel: w14 -> [w349]
          frame #0 {
            n160 = Wait (ms)(milliseconds to wait=w349) -> ()  [unwired: 1 out]
          }
        }
        n161 = flat-sequence {
          tunnel: w14 -> [w348]
          frame #0 {
            n162 = Wait (ms)(milliseconds to wait=w348) -> ()  [unwired: 1 out]
          }
        }
        n163 = flat-sequence {
          tunnel: w14 -> [w347]
          frame #0 {
            n164 = Wait (ms)(milliseconds to wait=w347) -> ()  [unwired: 1 out]
          }
        }
        n165 = flat-sequence {
          tunnel: w14 -> [w346]
          frame #0 {
            n166 = Wait (ms)(milliseconds to wait=w346) -> ()  [unwired: 1 out]
          }
        }
      }
      frame "Interval Change" {
        n167 = Build Array(u16 0 ("Handle"), u16 0 ("Handle")) -> (w383:u16[])
        n168 = call-poly "ble_write_by_handle.vi"("Connection Status"=w385, "Handle"=u16 12, "data (uint8array)"=w383, "COM Bluegiga in"=w372) -> ("error out"=w368:errorcluster)  [unwired: 6 in, 1 out]
        n169 = flat-sequence {
          tunnel: w360 -> [w396]
          tunnel: [w395] -> w369
          tunnel: w368 -> [w395]
          frame #0 {
            n170 = Wait (ms)(milliseconds to wait=w396) -> ()  [unwired: 1 out]
          }
        }
        n171 = Build Array(u16 0 ("Handle"), u16 0 ("Handle")) -> (w382:u16[])
        n172 = call-poly "ble_write_by_handle.vi"("Handle"=u16 16, "error in (no error)"=w369, "data (uint8array)"=w382, "COM Bluegiga in"=w372) -> ("error out"=w367:errorcluster)  [unwired: 6 in, 1 out]
        n173 = case shown="\"33ms\"" "Interval Time" {
          tunnel: [u8[] [74, 116, 10] u8[] [74, 116, 50] u8[] [74, 116, 66]] -> w370
          frame "10ms", Default {
          }
          frame "50ms" {
          }
          frame "33ms" {
          }
        }
        n174 = flat-sequence {
          tunnel: w360 -> [w394]
          tunnel: [w393] -> w366
          tunnel: w367 -> [w393]
          frame #0 {
            n175 = Wait (ms)(milliseconds to wait=w394) -> ()  [unwired: 1 out]
          }
        }
        n176 = call-poly "ble_write_by_handle.vi"("Handle"=u16 15, "error in (no error)"=w366, "data (uint8array)"=w370, "COM Bluegiga in"=w372) -> ("error out"=w365:errorcluster)  [unwired: 6 in, 1 out]
        n177 = flat-sequence {
          tunnel: u32 100 ("대기 시간(ms)") -> [w392]
          tunnel: [w391] -> w364
          tunnel: w365 -> [w391]
          frame #0 {
            n178 = Wait (ms)(milliseconds to wait=w392) -> ()  [unwired: 1 out]
          }
        }
        n179 = Build Array(u16 1 ("Handle"), u16 0 ("Handle")) -> (w376:u16[])
        n180 = call-poly "ble_write_by_handle.vi"("Handle"=u16 12, "error in (no error)"=w364, "data (uint8array)"=w376, "COM Bluegiga in"=w372) -> ("error out"=w363:errorcluster)  [unwired: 6 in, 1 out]
        n181 = flat-sequence {
          tunnel: w360 -> [w390]
          tunnel: [w389] -> w362
          tunnel: w363 -> [w389]
          frame #0 {
            n182 = Wait (ms)(milliseconds to wait=w390) -> ()  [unwired: 1 out]
          }
        }
        n183 = Build Array(u16 1 ("Handle"), u16 0 ("Handle")) -> (w377:u16[])
        n184 = call-poly "ble_write_by_handle.vi"("Handle"=u16 16, "error in (no error)"=w362, "data (uint8array)"=w377, "COM Bluegiga in"=w372) -> ("error out"=w361:errorcluster)  [unwired: 6 in, 1 out]
        n185 = flat-sequence {
          tunnel: w360 -> [w388]
          tunnel: [w387] -> _
          tunnel: w361 -> [w387]
          frame #0 {
            n186 = Wait (ms)(milliseconds to wait=w388) -> ()  [unwired: 1 out]
          }
        }
      }
      frame "Visa save" {
      }
    }
  }
  n187 = Wait (ms)(milliseconds to wait="Delay(ms)") -> ()  [unwired: 1 out]
